vi "Create DAQ.vi"(8 "error in (no error)":errorcluster, 9 "AO Channels":tag, 10 "AI Channels":tag, 11 "DAQ in":refnum<class "DAQ.lvclass">) -> (0 "error out":errorcluster, 3 "DAQ out":refnum<class "DAQ.lvclass">)   [LabVIEW 2016, in "DAQ.lvclass"]
uses:
  DAQ.lvclass
  C:/Program Files (x86)/National Instruments/LabVIEW 2016/vi.lib/JKI/JKI SMO/SMO/SMO.lvclass
  DAQ.lvclass/DAQ.ctl
  <vilib>/JKI/JKI SMO/SMO/SMO.lvclass
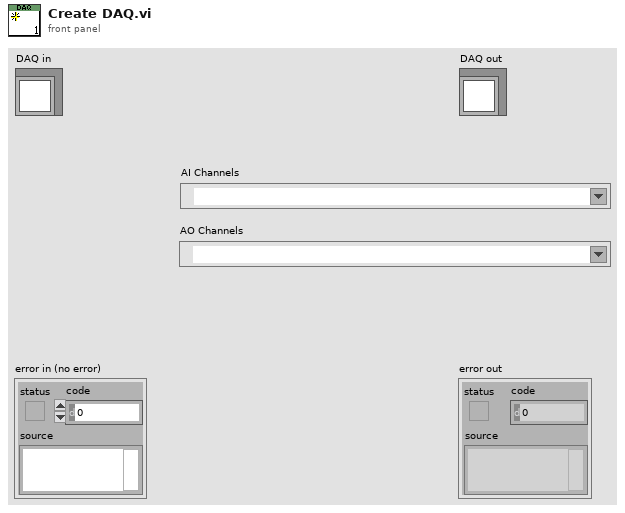
[diagram p1: front panel]
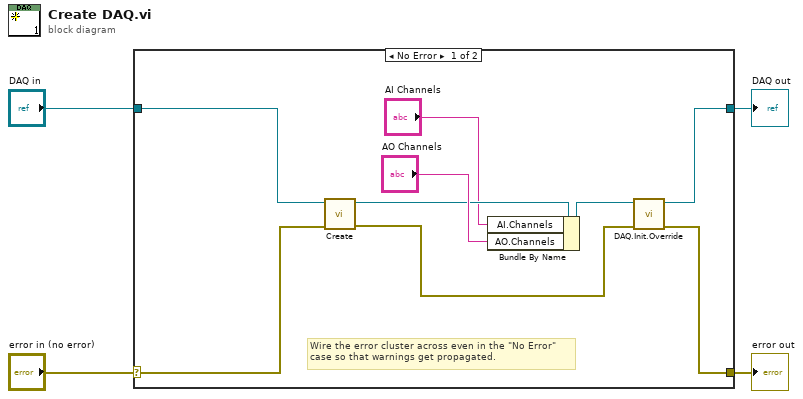
[diagram p0: block diagram]
diagram:
  n1 = case shown="No Error" "error in (no error)" {
    selector: "error in (no error)" -> [w12 w15]
    tunnel: [w7 w15] -> w3
    tunnel: [w9 w14] -> w1
    tunnel: "DAQ in" -> [w13 w14]
    frame No Error {
      # "Wire the error cluster across even in the \"No Error\"\ncase so that warnings get propagated."
      n2 = call <vilib>:"Create.vi"("error in (no error)"=w12, "SMO"=w13) -> ("error out"=w8:errorcluster, "SMO out"=w6:refnum<class "DAQ.lvclass">)  [unwired: 7 in, 1 out]
      n3 = Bundle By Name(cluster=w6, "AI.Channels"="AI Channels", "AO.Channels"="AO Channels") -> (w10:refnum<class "DAQ.lvclass">)
      n4 = call-dynamic "DAQ.Init.Override.vi"("error in (no error)"=w8, "DAQ in"=w10) -> ("error out"=w7:errorcluster, "DAQ out"=w9:refnum<class "DAQ.lvclass">)  [unwired: 8 in]
    }
    frame Error {
    }
  }
  "error out" <- w3
  "DAQ out" <- w1
